vi "wrt-fi-state.vi"(8 "error in (no error)":errorcluster, 10 "input.states":T1, 11 "frameInput in":refnum<class "bFrameIO.lvclass">) -> (0 "error out":errorcluster, 3 "frameInput out":refnum<class "bFrameIO.lvclass">)   [LabVIEW 2015, in "bFrameIO.lvclass"]
uses:
  bFrameIO.lvclass
  controls/input-states.ctl
  bFrameIO.lvclass/bFrameIO.ctl
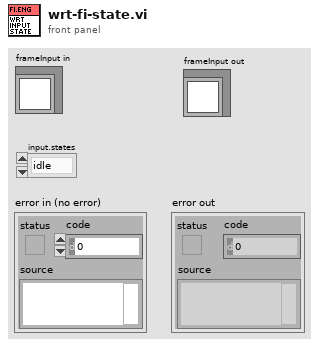
[diagram p1: front panel]
types:
  T1 = typedef "bFrameIO.lvclass/input-states.ctl" = enum16{"idle", "start", "run", "stop", "exit"}
  T2 = typedef "frameInput.lvclass/input.params.ctl" = cluster{"Interface":refnum<k21>, "CAN_Cluster":refnum<k21>, "input.states":T3, "baudrate":u32}
  T3 = typedef "frameInput.lvclass/input-states.ctl" = enum16{"idle", "start", "run", "stop", "exit"}
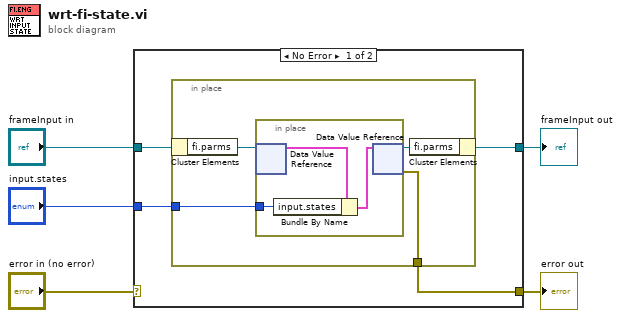
[diagram p0: block diagram]
diagram:
  n1 = case shown="No Error" "error in (no error)" {
    selector: "error in (no error)" -> [_ w17]
    tunnel: [w7 w17] -> w4
    tunnel: [w8 w18] -> w2
    tunnel: "frameInput in" -> [w9 w18]
    tunnel: "input.states" -> [w6 _]
    frame No Error {
      n2 = in-place {
        in-place-border: [w11] -> w7
        in-place-border: w6 -> [w10]
        n3 = in-place-cluster #1(w9) -> ("fi.parms"=w13:refnum<data-value>)
        n4 = in-place {
          in-place-border: w10 -> [w14]
          n5 = in-place-dvr #2(w13) -> (w16:T2)  [unwired: 1 out]
          n6 = Bundle By Name(cluster=w16, "input.states"=w14) -> (w15:T2)
          n7 = in-place-dvr #2(w15) -> (w12:refnum<data-value>, w11:errorcluster)
        }
        n8 = in-place-cluster #1("fi.parms"=w12) -> (w8:refnum<class "bFrameIO.lvclass">)
      }
    }
    frame Error {
    }
  }
  "error out" <- w4
  "frameInput out" <- w2
